vi "Connect.vi"(2 "error in (no error)":errorcluster caption="error in", 3 "Connection type":u16(ring) items=["USB", "RS232"], 4 "Com Port":refnum<visa-resource-name> caption="Com Port in") -> (0 "error out":errorcluster, 1 "VISA resource name out":refnum<visa-resource-name> caption="Com Port out")   [LabVIEW 2013]
doc: "Connects a Omicron Device to the Computer via a specific COM port.\n\nconnection type:\n\n- (0) USB: 500000baud\n- (1) RS232 : 57600 baud"
uses:
  <vilib>/Instr/_visa.llb/VISA Configure Serial Port (Instr).vi
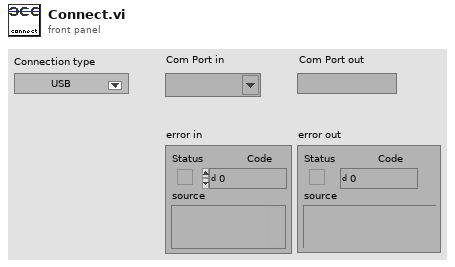
[diagram p1: front panel]
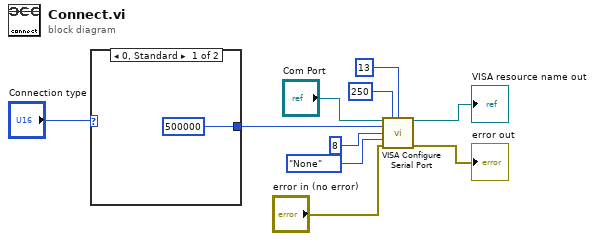
[diagram p0: block diagram]
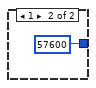
[diagram p2: hidden frame]
diagram:
  n1 = case shown="0, Standard" "Connection type" {
    tunnel: [u32 500000 ("baud rate (9600)") u32 57600 ("baud rate (9600)")] -> w2
    frame 0, Default {
    }
    frame 1 {
    }
  }
  n2 = call-poly "VISA Configure Serial Port"("VISA resource name"="Com Port", "timeout (10sec)"=u32 250, "termination char\n(0xA = '\\n' = LF)"=u8 13 ("termination char\n(0xA = '\\n' = LF)"), "baud rate (9600)"=w2, "data bits (8)"=u16 8, "parity (0:none)"=enum16{"None", "Odd", "Even", "Mark", "Space"}."None", "error in (no error)"="error in (no error)") -> ("VISA resource name out"=→"VISA resource name out":refnum<visa-resource-name>, "error out"=→"error out":errorcluster)  [unwired: 7 in]
